vi "ExitGui.vi"(11 "Message":string) -> (2 "ok":bool, 3 "ExitAction":T1=enum."Shut Down PC")   [LabVIEW 2016]
uses:
  Tools/Windows/Windows.ExitAction.ctl
  ExitGui.Action.ctl
  Tools/Translator/Translator.Global.vi
  Global/ApplicationGlobal.vi
panel:
  out "_loop":i32(ring)=4
  in  "ExitOption":u16(ring)=3 items=["Log off from PC", "Shut Down PC", "Reboot PC", "Close Program"]
  in  "CancelButton":bool
  in  "OKButton":bool
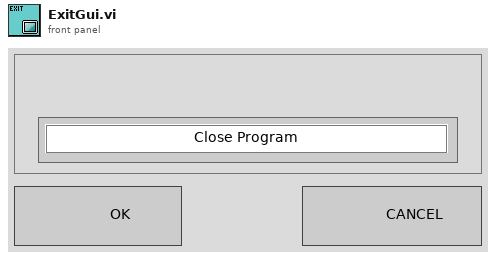
[diagram p1: front panel]
types:
  T1 = typedef "Windows.ExitAction.ctl" = enum16{"Log off from PC", "Shut Down PC", "Reboot PC", "Close Program"}
  T2 = typedef "ExitGui.Action.ctl" = enum32{"idle", "constructor", "destructor", "--- ExitGUI ---"}
  T3 = typedef "LVPositionTypeDef.ctl" = cluster{"Left":i32, "Top":i32}
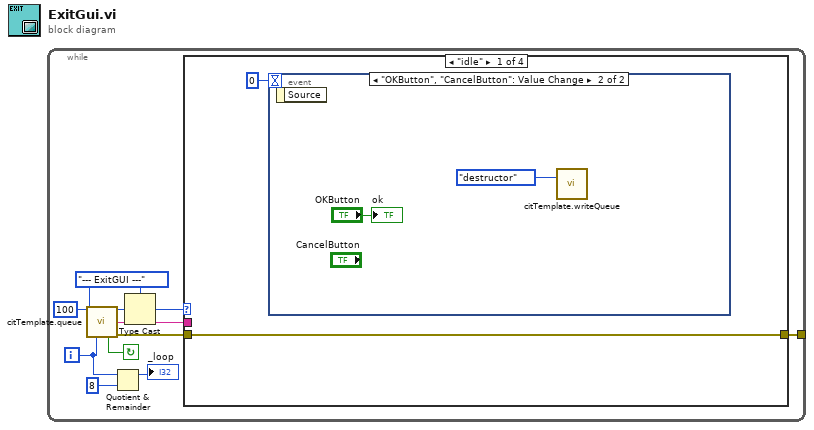
[diagram p0: block diagram]
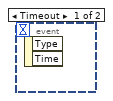
[diagram p2: hidden frame]
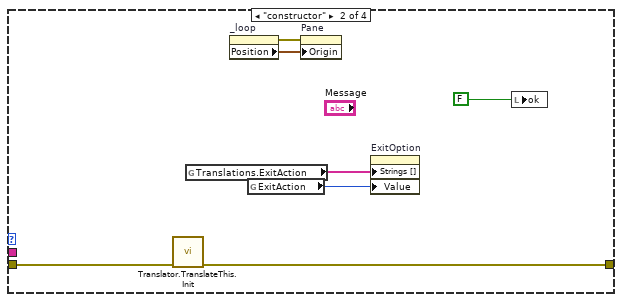
[diagram p3: hidden frame]
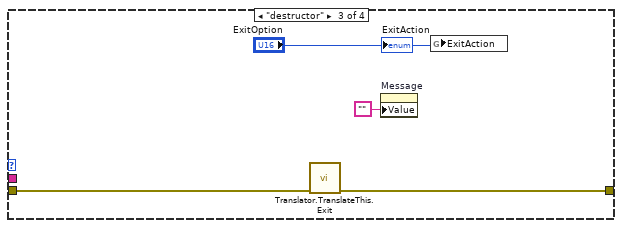
[diagram p4: hidden frame]
diagram:
  n1 = while {
    tunnel: [w1] -> _
    i -> [w2]
    stop <- w11 continue-if-true
    w5 = ExitGui.Action."--- ExitGUI ---" ("Action")
    n2 = call "citTemplate.queue.vi"("ms timeout (250 ms)"=100, "event enum"=w5, "iteration (-1)"=w2) -> ("event out"=w9:u32, "(flatten) data out"=w6:string, "continue"=w11:bool, "error out"=w7:errorcluster)  [unwired: 2 in, 7 out]
    n3 = Quotient & Remainder(x=w2, y=8) -> (x-y*floor(x/y)=→"_loop":i32)  [unwired: 1 out]
    n4 = Type Cast(type=w5, x=w9) -> (*(type *) &x=w8:T2)
    n5 = case shown="\"idle\"" w8 {
      tunnel: w7 -> [w12 w17 w24 w27]
      tunnel: w6 -> [_ _ _ _]
      tunnel: [w12 w16 w23 w27] -> w1
      frame "idle" {
        n6 = event shown="[1] \"OKButton\", \"CancelButton\": Value Change" {
          selector: _ -> [_ _]
          dyn-events: _ -> [_ _]
          timeout: 0 -> [_ _]
          event Timeout {
            n7 = event-data() -> ()  [unwired: 3 out]
          }
          event "OKButton", "CancelButton": Value Change {
            n8 = event-data() -> ()  [unwired: 2 out]
            n9 = call "citTemplate.writeQueue.vi"("event in (if not connected:all statemachine with data event)"=ExitGui.Action."destructor" ("Action")) -> ()  [unwired: 14 in, 1 out]
            "ok" <- "OKButton"
          }
        }
      }
      frame "constructor" {
        n10 = call "Translator.TranslateThis.Init.vi"("error in"=w17) -> ("error out"=w16:errorcluster)  [unwired: 10 in]
        n11 = global read "Translator.Global.vi" "Translations.ExitAction"() -> (w19:string[])
        n12 = property on="_loop" class="Ring (strict)"() -> (error out=w20:errorcluster, "Position"=w21:T3)  [unwired: 2 in, 1 out]
        n13 = global read "ApplicationGlobal.vi" "ExitAction"() -> (w18:T1)
        n14 = property on="Pane" class="Pane"(error in=w20, "Origin"=w21) -> ()  [unwired: 1 in, 2 out]
        n15 = property on="ExitOption" class="Ring (strict)"("Strings []"=w19, "Value"=w18) -> ()  [unwired: 2 in, 2 out]
        n16 = local write "ok"(FALSE ("_b_ok")) -> ()
      }
      frame "destructor" {
        n17 = call "Translator.TranslateThis.Exit.vi"("error in"=w24) -> ("error out"=w23:errorcluster)  [unwired: 10 in]
        n18 = property on="Message" class="Str"("Value"="") -> ()  [unwired: 2 in, 2 out]
        n19 = global write "ApplicationGlobal.vi" "ExitAction"("ExitOption") -> ()
        "ExitAction" <- "ExitOption"
      }
      frame "--- ExitGUI ---" {
      }
    }
  }
